vi "Fibonacci_Series.vi"() -> ()   [LabVIEW 2019]
panel:
  out "Array":dbl[](array[numeric])
  in  "Numeric":i32
  # "Fibonacci Series"
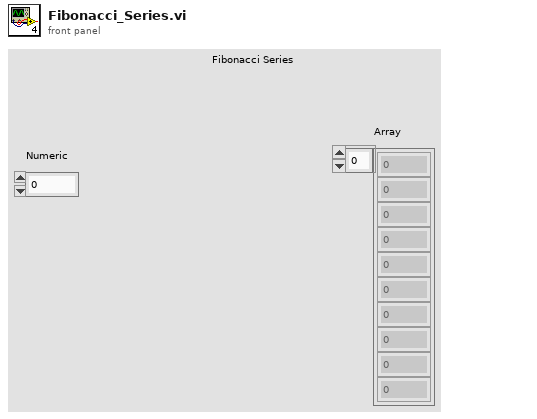
[diagram p1: front panel]
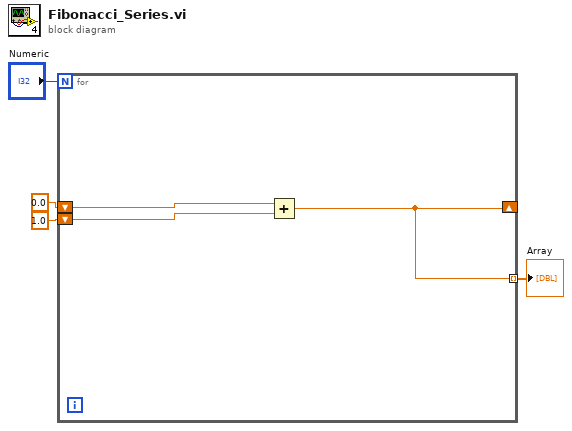
[diagram p0: block diagram]
diagram:
  n1 = for {
    N: "Numeric" -> [_]
    shift-right: [w5] -> _
    shift-left: 0.0 -> [w7]
    shift-left: 1.0 -> [w6]
    tunnel: [w5] -> w1 mode=indexing
    n2 = Add(x=w7, y=w6) -> (x+y=w5:dbl)
  }
  "Array" <- w1
